vi "file_exist.vi"(1 "File path name input":path) -> (0 "File exist?":bool)   [LabVIEW 2017]
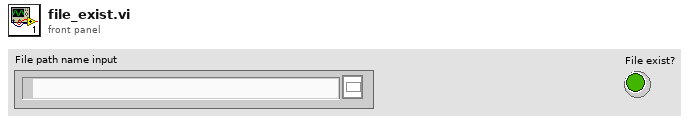
[diagram p1: front panel]
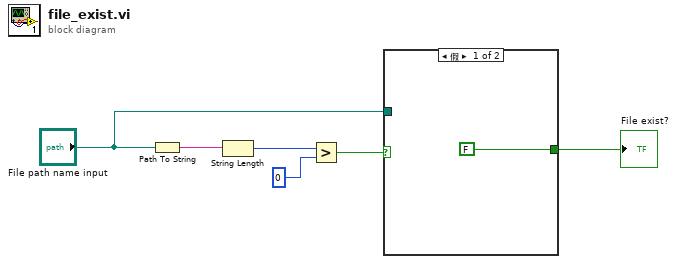
[diagram p0: block diagram]
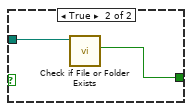
[diagram p2: hidden frame]
diagram:
  n1 = Path To String(path="File path name input") -> (string=w6:string)
  n2 = String Length(string=w6) -> (length=w5:i32)
  n3 = Greater?(x=w5, y=0) -> (0:w3:bool)
  n4 = case shown="假" w3 {
    tunnel: [FALSE w8] -> w2
    tunnel: "File path name input" -> [_ w9]
    frame False {
    }
    frame True {
      n5 = call <vilib>:"Check if File or Folder Exists.vi"("path"=w9) -> ("file or folder exists?"=w8:bool)  [unwired: 8 in, 2 out]
    }
  }
  "File exist?" <- w2
